vi "niFpgaDsp48eSimTemplate.vi"(0 "a/acin":fxp<+/-,30,30>, 1 "b/bcin":fxp<+/-,18,18>, 2 "pcin":fxp<+/-,48,48>, 3 "c":fxp<+/-,48,48>, 4 "carryinsel":fxp<+,3,3> format="%.0b", 5 "opmode":fxp<+,7,7> format="%.0b", 6 "alumode":fxp<+,4,4> format="%.0b", 7 "carryin":bool, 8 "resets":T9, 9 "carrycascin":bool, 10 "enables":T10={"cea1"=TRUE, "cea2"=TRUE, "cead"=TRUE, "cealumode"=TRUE, "ceb1"=TRUE, "ceb2"=TRUE, "cec"=TRUE, "cecarryin"=TRUE, "cectrl"=TRUE, "ced"=TRUE, "ceinmode"=TRUE, "cem"=TRUE, "cemultcarryin"=TRUE, "cep"=TRUE}, 11 "multsignin":bool, 12 "simulation state":T1={"type"=enum."DSP48E", "Functions"={"control signal settings"=enum."Show Terminals", "Multiplier mode"=enum."dynamic", "Logic unit mode"=enum."one 48-bit", "Use pre-adder"=FALSE}, "Pattern detection"={"Use pattern detect"=FALSE, "Selet pattern"=enum."pattern constant", "Pattern constant"=0, "Select mask"=enum."mask constant", "Mask constant"=0, "Autoreset pattern detect"=enum."no reset"}, "Registers"={"Number of a registers"=0, "Number of b registers"=0, "Registers from a to acout"=0, "Registers from b to bcout"=0, "ad register"=FALSE, "alumode register"=FALSE, "c register"=FALSE, "carryin register"=FALSE, "carryinsel register"=FALSE, "d register"=FALSE, "inmode register"=FALSE, "m register"=FALSE, "multcarryin register"=FALSE, "opmode register"=FALSE, "p register"=FALSE}} {"Pattern detection"."Mask constant" format="%012x"; "Pattern detection"."Pattern constant" format="%012x"}, 13 "d":fxp<+/-,25,25>, 15 "inmode":fxp<+,5,5> format="%.0b") -> (16 "acout":fxp<+/-,30,30>, 18 "bcout":fxp<+/-,18,18>, 20 "p":fxp<+/-,48,48>, 21 "carryout":fxp<+,4,4>, 22 "carrycascout":bool, 23 "multsignout":bool, 24 "patterndetect":bool, 25 "patternbdetect":bool, 26 "overflow":bool, 27 "underflow":bool)   [LabVIEW 2017]
uses:
  <vilib>/rvi/FXPMathLib/basic elements/DSP48E/simVIs/niFpgaDsp48eEnables.ctl
  <vilib>/rvi/FXPMathLib/basic elements/DSP48E/simVIs/niFpgaDsp48eResets.ctl
  <vilib>/rvi/FXPMathLib/basic elements/DSP48E/simVIs/niFpgaDsp48eSimulationState.ctl
  <vilib>/rvi/FXPMathLib/basic elements/DSP48E/subVIs/niFpgaDsp48eType.ctl
  <vilib>/rvi/FXPMathLib/basic elements/DSP48E/subVIs/niFpgaDsp48eAlumodeOpmodeCarryinselState.ctl
  <vilib>/rvi/FXPMathLib/basic elements/DSP48E/subVIs/niFpgaDsp48eUseMultiplierState.ctl
  <vilib>/rvi/FXPMathLib/basic elements/DSP48E/subVIs/niFpgaDsp48eLogicUnitModeState.ctl
  <vilib>/rvi/FXPMathLib/basic elements/DSP48E/subVIs/niFpgaDsp48eSelectPatternState.ctl
  <vilib>/rvi/FXPMathLib/basic elements/DSP48E/subVIs/niFpgaDsp48eSelectMaskState.ctl
  <vilib>/rvi/FXPMathLib/basic elements/DSP48E/subVIs/niFpgaDsp48eAutoresetState.ctl
  <vilib>/rvi/FXPMathLib/basic elements/DSP48E/simVIs/niFpgaDsp48eRegisters.ctl
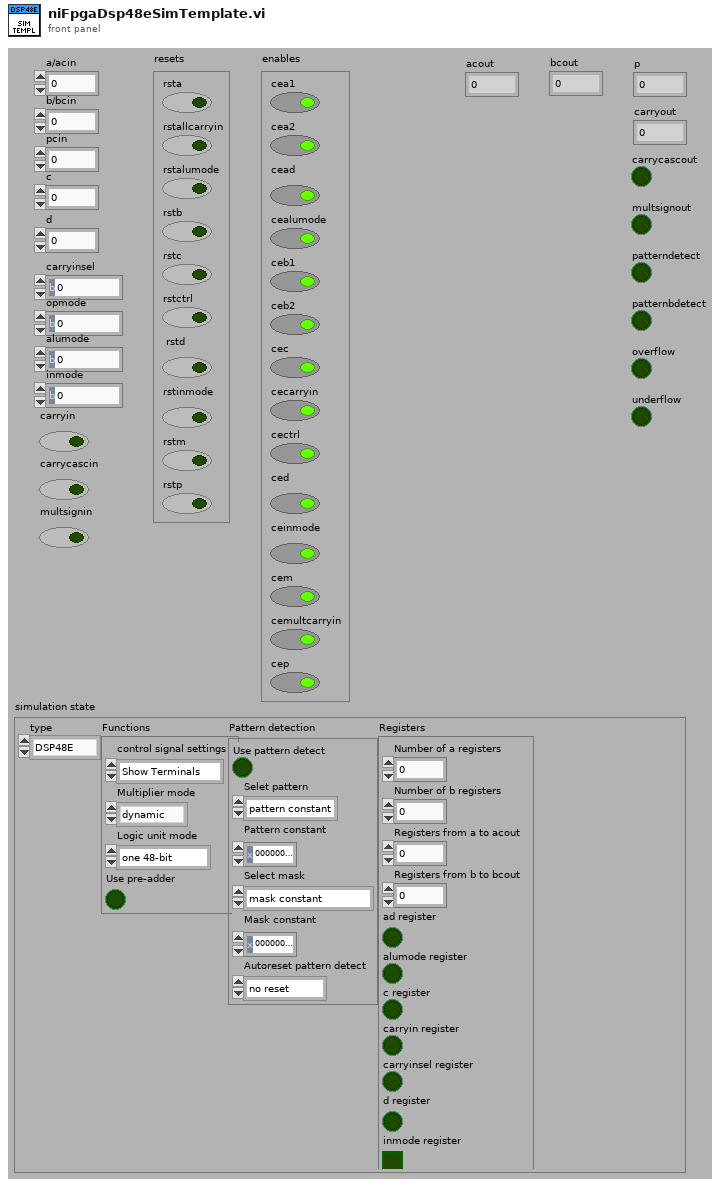
[diagram p1: front panel]
types:
  T1 = typedef "niFpgaDsp48eSimulationState.ctl" = cluster{"type":T2, "Functions":cluster{"control signal settings":T3, "Multiplier mode":T4, "Logic unit mode":T5, "Use pre-adder":bool}, "Pattern detection":cluster{"Use pattern detect":bool, "Selet pattern":T6, "Pattern constant":u64, "Select mask":T7, "Mask constant":u64, "Autoreset pattern detect":T8}, "Registers":cluster{"Number of a registers":u8, "Number of b registers":u8, "Registers from a to acout":u8, "Registers from b to bcout":u8, "ad register":bool, "alumode register":bool, "c register":bool, "carryin register":bool, "carryinsel register":bool, "d register":bool, "inmode register":bool, "m register":bool, "multcarryin register":bool, "opmode register":bool, "p register":bool}}
  T2 = typedef "niFpgaDsp48eType.ctl" = enum16{"DSP48E", "DSP48E1"}
  T3 = typedef "niFpgaDsp48eAlumodeOpmodeCarryinselState.ctl" = enum16{"Show Terminals", "Arithmetic", "Logic"}
  T4 = typedef "niFpgaDsp48eUseMultiplierState.ctl" = enum16{"none", "multiply", "dynamic"}
  T5 = typedef "niFpgaDsp48eLogicUnitModeState.ctl" = enum16{"one 48-bit", "two 24-bit", "four 12-bit"}
  T6 = typedef "niFpgaDsp48eSelectPatternState.ctl" = enum16{"pattern constant", "c reg data"}
  T7 = typedef "niFpgaDsp48eSelectMaskState.ctl" = enum16{"mask constant", "c reg data", "(not (c reg data))<<1", "(not (c reg data))<<2"}
  T8 = typedef "niFpgaDsp48eAutoresetState.ctl" = enum16{"no reset", "reset match", "reset not match"}
  T9 = typedef "niFpgaDsp48eResets.ctl" = cluster{"rsta":bool, "rstallcarryin":bool, "rstalumode":bool, "rstb":bool, "rstc":bool, "rstctrl":bool, "rstd":bool, "rstinmode":bool, "rstm":bool, "rstp":bool}
  T10 = typedef "niFpgaDsp48eEnables.ctl" = cluster{"cea1":bool, "cea2":bool, "cead":bool, "cealumode":bool, "ceb1":bool, "ceb2":bool, "cec":bool, "cecarryin":bool, "cectrl":bool, "ced":bool, "ceinmode":bool, "cem":bool, "cemultcarryin":bool, "cep":bool}
  T11 = typedef "niFpgaDsp48eRegisters.ctl" = cluster{"a register 1":fxp<+/-,30,30>, "a register 2":fxp<+/-,30,30>, "b register 1":fxp<+/-,18,18>, "b register 2":fxp<+/-,18,18>, "c register":fxp<+/-,48,48>, "d register":fxp<+/-,25,25>, "ad register":fxp<+/-,27,27>, "m register":fxp<+/-,45,45>, "opmode register":fxp<+,7,7>, "alumode register":fxp<+,4,4>, "carryinsel register":fxp<+,3,3>, "inmode register":fxp<+,5,5>, "carryin register":bool, "multcarryin register":bool, "p registers":fxp<+/-,48,48>, "carryout register":fxp<+,4,4>, "carrycascout register":bool, "multsignout register":bool, "patterndetect register":bool, "patternbdetect register":bool, "patterndetect register 2":bool, "patternbdetect register 2":bool}
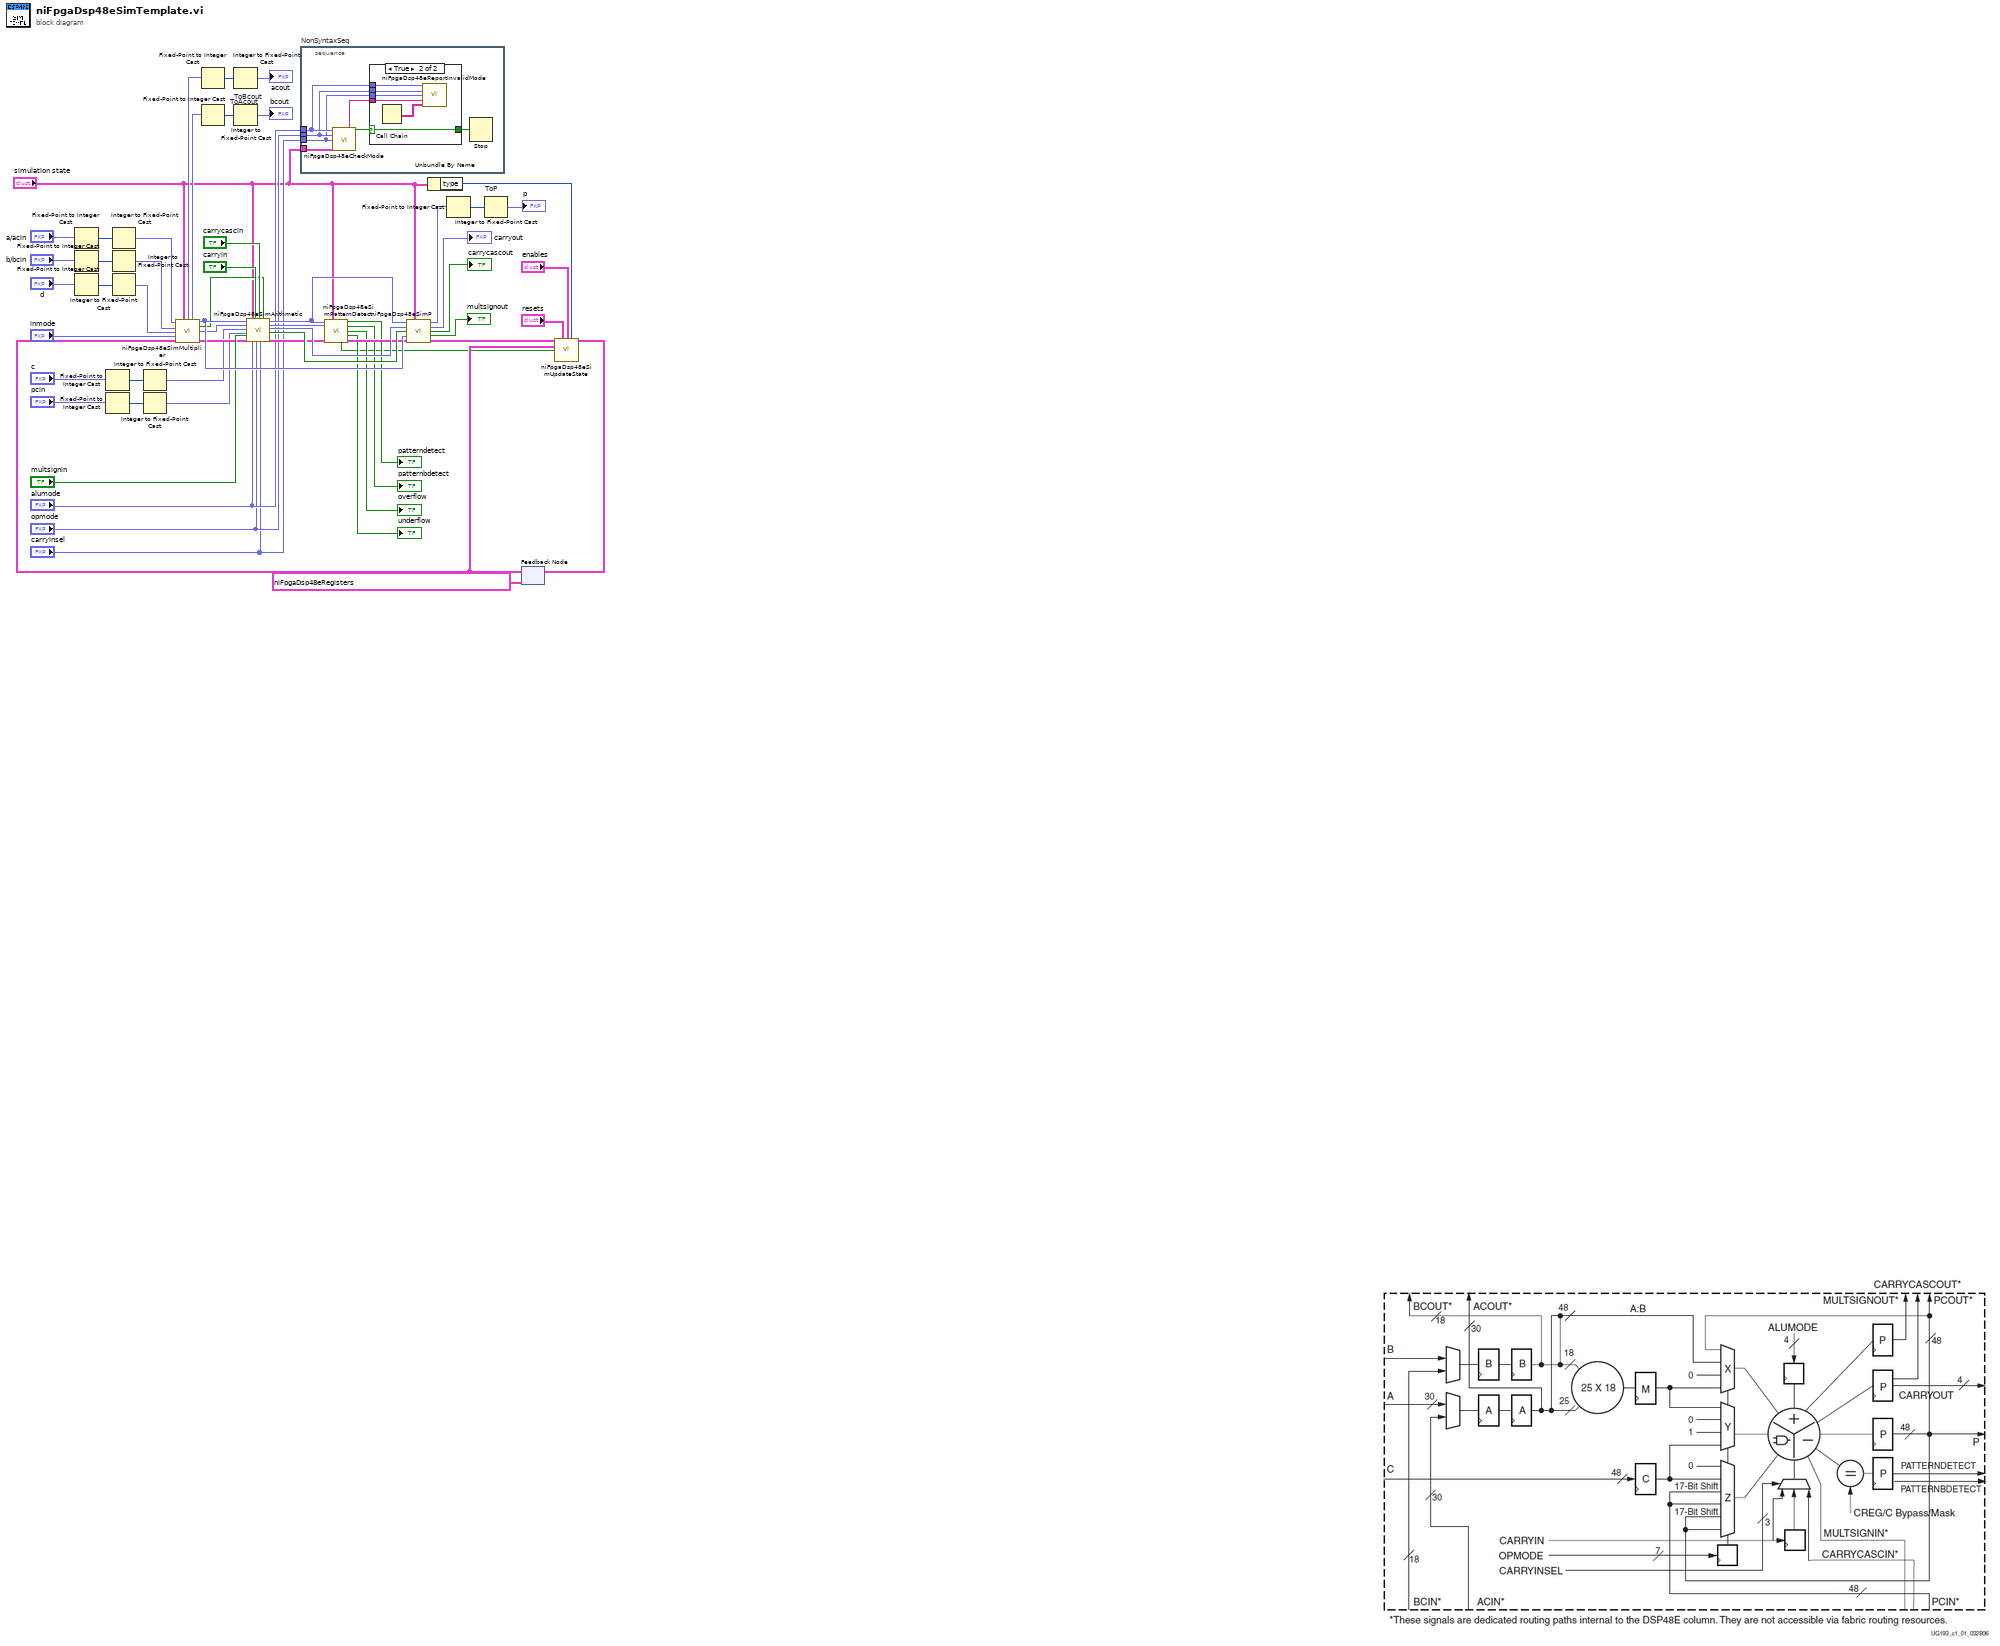
[diagram p0: block diagram]
diagram:
  n1 = Fixed-Point to Integer Cast(1:"a/acin") -> (0:w24:i32)
  n2 = Fixed-Point to Integer Cast(1:"b/bcin") -> (0:w23:i32)
  n3 = Fixed-Point to Integer Cast(1:"d") -> (0:w21:i32)
  n4 = Fixed-Point to Integer Cast(1:"c") -> (0:w15:i64)
  n5 = Fixed-Point to Integer Cast(1:"pcin") -> (0:w16:i64)
  n6 = Integer to Fixed-Point Cast(integer=w24) -> (fixed-point=w22:fxp<+/-,30,30>)  [unwired: 1 in]
  n7 = Integer to Fixed-Point Cast(integer=w23) -> (fixed-point=w19:fxp<+/-,18,18>)  [unwired: 1 in]
  n8 = Integer to Fixed-Point Cast(integer=w21) -> (fixed-point=w17:fxp<+/-,25,25>)  [unwired: 1 in]
  n9 = Integer to Fixed-Point Cast(integer=w15) -> (fixed-point=w13:fxp<+/-,48,48>)  [unwired: 1 in]
  n10 = Integer to Fixed-Point Cast(integer=w16) -> (fixed-point=w11:fxp<+/-,48,48>)  [unwired: 1 in]
  n11 = stacked-sequence "NonSyntaxSeq" {
    tunnel: "alumode" -> [w61]
    tunnel: "opmode" -> [w60]
    tunnel: "carryinsel" -> [w59]
    tunnel: "simulation state" -> [w62]
    frame #0 {
      n12 = call <vilib>:"niFpgaDsp48eCheckMode.vi"("alumode"=w61, "opmode"=w60, "carryinsel"=w59, "simulation state"=w62) -> ("error information"=w64:string, "invalid configuration"=w63:bool)  [unwired: 10 in]
      n13 = case shown="True" w63 {
        selector: w63 -> [_ w65]
        tunnel: w64 -> [_ w67]
        tunnel: w61 -> [_ w70]
        tunnel: w60 -> [_ w69]
        tunnel: w59 -> [_ w68]
        tunnel: [_ w65] -> w58
        frame False {
        }
        frame True {
          n14 = Call Chain() -> (call chain=w66:string[])
          n15 = call <vilib>:"niFpgaDsp48eReportInvalidMode.vi"("alumode"=w70, "opmode"=w69, "carryinsel"=w68, "error information"=w67, "call chain"=w66) -> ()  [unwired: 11 in]
        }
      }
      n16 = Stop(stop? (T)=w58) -> ()
    }
  }
  n17 = Unbundle By Name("simulation state") -> ("type"=w30:T2)
  n18 = feedback #1(T11 {"a register 1"=0.0, "a register 2"=0.0, "b register 1"=0.0, "b register 2"=0.0, "c register"=0.0, "d register"=0.0, "ad register"=0.0, "m register"=0.0, "opmode register"=0.0, "alumode register"=0.0, "carryinsel register"=0.0, "inmode register"=0.0, "carryin register"=FALSE, "multcarryin register"=FALSE, "p registers"=0.0, "carryout register"=0.0, "carrycascout register"=FALSE, "multsignout register"=FALSE, "patterndetect register"=FALSE, "patternbdetect register"=FALSE, "patterndetect register 2"=FALSE, "patternbdetect register 2"=FALSE} ("Simulation state out")) -> (w56:T11)
  n19 = call <vilib>:"niFpgaDsp48eSimMultiplier.vi"("a/acin"=w22, "state"="simulation state", "b/bcin"=w19, "d"=w17, "inmode"="inmode", "register state"=w56) -> ("acout"=w6:fxp<+/-,30,30>, "bcout"=w2:fxp<+/-,18,18>, "multiplier out"=w49:fxp<+/-,45,45>, "multcarryin"=w34:bool, "a:b"=w33:fxp<+/-,48,48>, "register state next"=w35:T11)  [unwired: 4 in]
  n20 = Fixed-Point to Integer Cast(1:w6) -> (0:w7:i32)
  n21 = Fixed-Point to Integer Cast(1:w2) -> (0:w4:i32)
  n22 = Integer to Fixed-Point Cast "ToAcout"(integer=w7) -> (fixed-point=→"acout":fxp<+/-,30,30>)  [unwired: 1 in]
  n23 = Integer to Fixed-Point Cast "ToBcout"(integer=w4) -> (fixed-point=→"bcout":fxp<+/-,18,18>)  [unwired: 1 in]
  n24 = call <vilib>:"niFpgaDsp48eSimArithmetic.vi"("multiplier out"=w49, "a:b"=w33, "c"=w13, "pcin"=w11, "multsignin"="multsignin", "register state"=w35, "simulation state"="simulation state", "alumode"="alumode", "carryin"="carryin", "opmode"="opmode", "carrycascin"="carrycascin", "carryinsel"="carryinsel", "multicarryin"=w34) -> ("p"=w46:fxp<+/-,48,48>, "c register out"=w39:fxp<+/-,48,48>, "carryout"=w47:fxp<+,4,4>, "carrycascout"=w48:bool, "register state next"=w40:T11)  [unwired: 2 in]
  n25 = call <vilib>:"niFpgaDsp48eSimPatternDetect.vi"("p"=w46, "simulation state"="simulation state", "c"=w39, "register state"=w40) -> ("patterndetect"=→"patterndetect":bool, "patternbdetect"=→"patternbdetect":bool, "overflow"=→"overflow":bool, "underflow"=→"underflow":bool, "autoreset p registers"=w26:bool, "register state next"=w45:T11)  [unwired: 6 in]
  n26 = call <vilib>:"niFpgaDsp48eSimP.vi"("p"=w46, "simulation state"="simulation state", "carryout"=w47, "carrycascout"=w48, "multiplier out"=w49, "register state"=w45) -> ("p out"=w9:fxp<+/-,48,48>, "carryout out"=→"carryout":fxp<+,4,4>, "carrycascout out"=→"carrycascout":bool, "multsignout out"=→"multsignout":bool, "register state next"=w53:T11)  [unwired: 5 in]
  n27 = Fixed-Point to Integer Cast(1:w9) -> (0:w10:i64)
  n28 = Integer to Fixed-Point Cast "ToP"(integer=w10) -> (fixed-point=→"p":fxp<+/-,48,48>)  [unwired: 1 in]
  n29 = call <vilib>:"niFpgaDsp48eSimUpdateState.vi"("register state"=w53, "resets"="resets", "enables"="enables", "type"=w30, "original register state"=w56, "autoreset p registers"=w26) -> ("register state next"=w57:T11)  [unwired: 9 in]
  n30 = feedback-in #1(w57) -> ()
